vi "scanWaveGen.vi"(6 "overScanBlanking":bool, 8 "singleDirScan":bool, 9 "numRoundingPts":i32, 10 "scanWaveForm":T2(ring), 11 "numPts":dbl) -> (2 "blankingParams":T1, 3 "outWave":dbl[](array[numeric]))   [LabVIEW 2016]
uses:
  <vilib>/measure/NI_MABase.lvlib
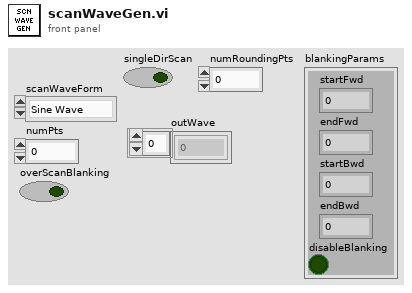
[diagram p1: front panel]
types:
  T1 = cluster{"startFwd":u16, "endFwd":u16, "startBwd":u16, "endBwd":u16, "disableBlanking":bool}
  T2 = enum16{"Sine Wave", "Triangle Wave", "Square Wave", "Sawtooth Wave", "Rounded Triangle"}
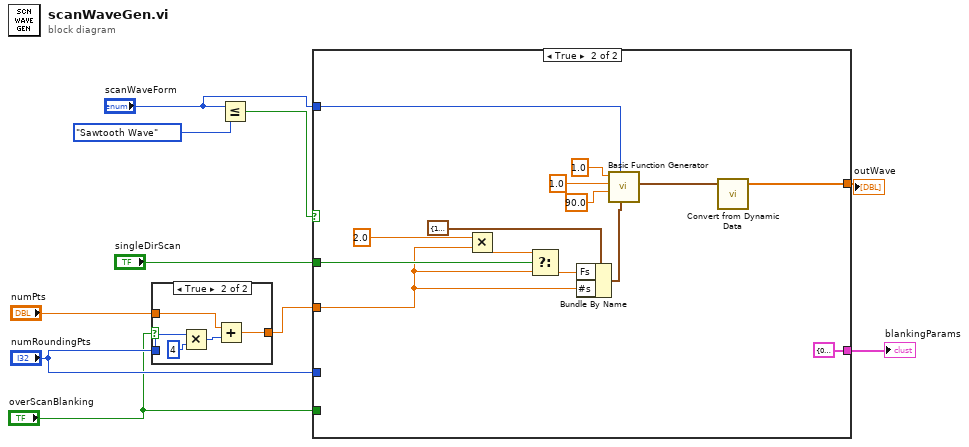
[diagram p0: block diagram]
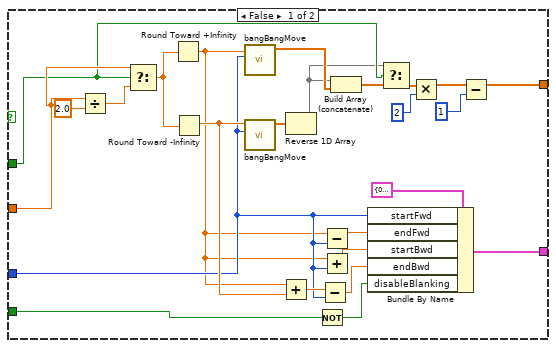
[diagram p3: hidden frame]
diagram:
  n1 = case shown="True" "overScanBlanking" {
    tunnel: "numRoundingPts" -> [_ w16]
    tunnel: "numPts" -> [w11 w13]
    tunnel: [w11 w12] -> w3
    frame False {
    }
    frame True {
      n2 = Multiply(x=w16, y=4) -> (x*y=w14:i32)
      n3 = Add(x=w13, y=w14) -> (x+y=w12:dbl)
    }
  }
  n4 = Less Or Equal?(x="scanWaveForm", y=T2."Sawtooth Wave") -> (x <= y?=w8:bool)
  n5 = case shown="True" w8 {
    tunnel: "singleDirScan" -> [w29 w48]
    tunnel: w3 -> [w32 w47]
    tunnel: "scanWaveForm" -> [_ w44]
    tunnel: "numRoundingPts" -> [w22 _]
    tunnel: [w37 w43] -> w7
    tunnel: "overScanBlanking" -> [w20 _]
    tunnel: [w18 T1 {"startFwd"=0, "endFwd"=0, "startBwd"=0, "endBwd"=0, "disableBlanking"=TRUE} ("fastBlanking")] -> w1
    frame False {
      n6 = Divide(x=w32, y=2.0) -> (x/y=w33:dbl)
      n7 = Select(t=w32, s=w29, f=w33) -> (s? t:f=w31:dbl)
      n8 = Round Toward +Infinity(x=w31) -> (ceil(x): smallest int >= x=w17:dbl)
      n9 = Round Toward -Infinity(1:w31) -> (0:w24:dbl)
      n10 = call "bangBangMove.vi"("numRoundingPts"=w22, "numPts"=w17) -> ("roundedHalfTriangle"=w35:dbl[])  [unwired: 9 in]
      n11 = call "bangBangMove.vi"("numRoundingPts"=w22, "numPts"=w24) -> ("roundedHalfTriangle"=w41:dbl[])  [unwired: 9 in]
      n12 = Add(x=w17, y=w24) -> (x+y=w23:dbl)
      n13 = Reverse 1D Array(array=w41) -> (reversed array=w28:dbl[])
      n14 = Not(x=w20) -> (.not. x?=w19:bool)
      n15 = Subtract(x=w23, y=w22) -> (x-y=w21:dbl)
      n16 = Subtract(x=w17, y=w22) -> (x-y=w26:dbl)
      n17 = Add(x=w17, y=w22) -> (x+y=w25:dbl)
      n18 = Build Array (concatenate)(w28, w35) -> (w40:dbl[])
      n19 = Bundle By Name(cluster=T1 {"startFwd"=0, "endFwd"=0, "startBwd"=0, "endBwd"=0, "disableBlanking"=FALSE} ("fastBlanking"), "startFwd"=w22, "endFwd"=w26, "startBwd"=w25, "endBwd"=w21, "disableBlanking"=w19) -> (w18:T1)
      n20 = Select(t=w28, s=w29, f=w40) -> (s? t:f=w30:dbl[])
      n21 = Multiply(x=w30, y=2) -> (x*y=w39:dbl[])
      n22 = Subtract(x=w39, y=1) -> (x-y=w37:dbl[])
    }
    frame True {
      n23 = Multiply(x=2.0, y=w47) -> (x*y=w46:dbl)
      n24 = Select(t=w46, s=w48, f=w47) -> (s? t:f=w49:dbl)
      n25 = Bundle By Name(cluster=cluster{"Fs":dbl, "#s":dbl} {"Fs"=1000.0, "#s"=1000.0} ("sampling info"), "Fs"=w49, "#s"=w47) -> (w53:cluster{"Fs":dbl, "#s":dbl})
      n26 = call <vilib>:"Basic Function Generator.vi"("sampling info"=w53, "signal type"=w44, "phase"=90.0, "amplitude"=1.0, "frequency"=1.0) -> ("signal out"=w50:waveform(dbl))  [unwired: 4 in, 2 out]
      n27 = call "Convert from Dynamic Data"("Dynamic Data Type"=w50) -> ("Array"=w43:dbl[])  [unwired: 3 in]
    }
  }
  "outWave" <- w7
  "blankingParams" <- w1
